vi "AB_Paths_To_Strings.vi"(10 "paths":path[](array[path])) -> (2 "strings":string[](array[string]))   [LabVIEW 2020]
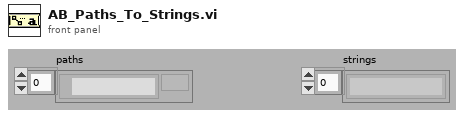
[diagram p1: front panel]
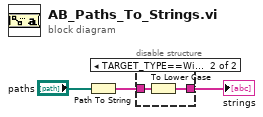
[diagram p0: block diagram]
diagram:
  n1 = Path To String(path="paths") -> (string=w3:string[])
  n2 = disable-structure shown="TARGET_TYPE==Windows" {
    disable-tunnel: w3 -> [w4 w6]
    disable-tunnel: [w4 w5] -> w2
    frame condition #0 {
    }
    frame condition #1 (active) {
      n3 = To Lower Case(string=w6) -> (all lower case string=w5:string[])
    }
  }
  "strings" <- w2
